vi "GET Experimental Data Save VI Reference.vi"() -> (0 "Experimental Data Save VI Reference":refnum<vi>)   [LabVIEW 2013]
uses:
  Action.ctl
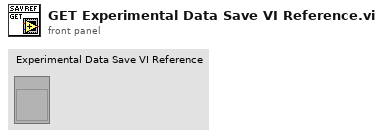
[diagram p1: front panel]
types:
  T1 = typedef "Action.ctl" = enum16{"GET", "PUT", "DELETE"}
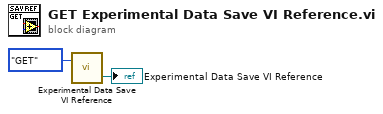
[diagram p0: block diagram]
diagram:
  n1 = call "Experimental Data Save VI Reference.vi"("Action"=Action."GET") -> ("Output"=→"Experimental Data Save VI Reference":refnum<vi>)  [unwired: 2 in]
